vi "Fill Wfm Attribute.vi"(8 "Error In":errorcluster, 9 "Description":string="Power", 10 "Unit":string="W", 11 "Channel Name":string="NI_ChannelName") -> (0 "Error Out":errorcluster, 3 "Wfm Attributes":variant)   [LabVIEW 2016, in "KIT-QA.lvlib" / "KIT-QA.lvclass"]
doc: "Fill waveform attribute variant."
uses:
  KIT-QA.lvclass
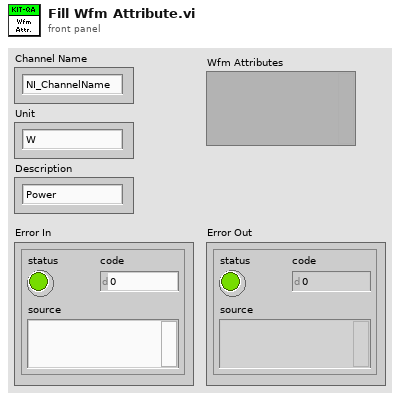
[diagram p1: front panel]
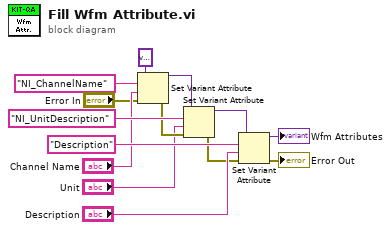
[diagram p0: block diagram]
diagram:
  n1 = Set Variant Attribute(Variant=variant ("attributes"), name="NI_ChannelName", value="Channel Name", error in="Error In") -> (Variant out=w9:variant, error out=w8:errorcluster)  [unwired: 1 out]
  n2 = Set Variant Attribute(Variant=w9, name="NI_UnitDescription", value="Unit", error in=w8) -> (Variant out=w13:variant, error out=w4:errorcluster)  [unwired: 1 out]
  n3 = Set Variant Attribute(Variant=w13, name="Description", value="Description", error in=w4) -> (Variant out=→"Wfm Attributes":variant, error out=→"Error Out":errorcluster)  [unwired: 1 out]
